vi "DCV_MultChannel.vi"(8 "Error In":errorcluster, 9 "End channel":string="116", 10 "Start channel":string="101", 11 "VISA resource name":refnum<visa-resource-name>="COM5") -> (0 "Error Out":errorcluster, 2 "testlist":dbl[](array[numeric])=[1.33831, 1.33831, 1.33831, 1.33831, 1.3383, 1.3383, 1.3383, 1.3383, 1.33829, 1.33829, 1.33829, 1.33829, 1.33828, 1.33828, 1.33828, 1.33828], 3 "VISA resource name out":refnum<visa-resource-name>="COM5")   [LabVIEW 2013]
uses:
  <vilib>/Utility/error.llb/whitespace.ctl
panel:
  out "number":dbl=1.33828
  out "read buffer":string="SCAN OK\n"
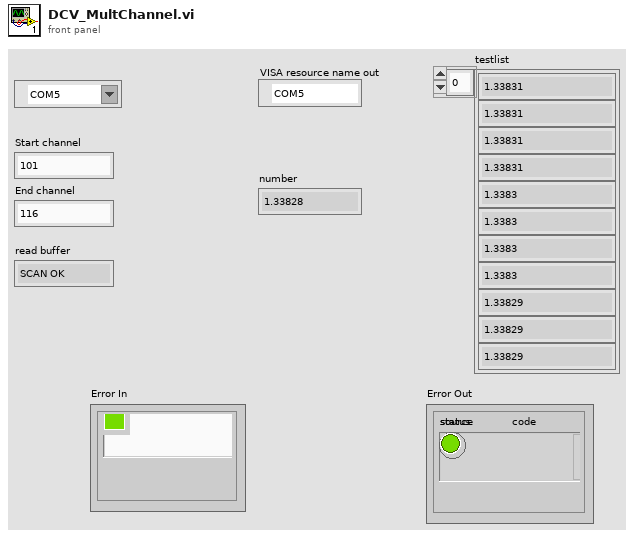
[diagram p1: front panel]
types:
  T1 = typedef "whitespace.ctl" = u16
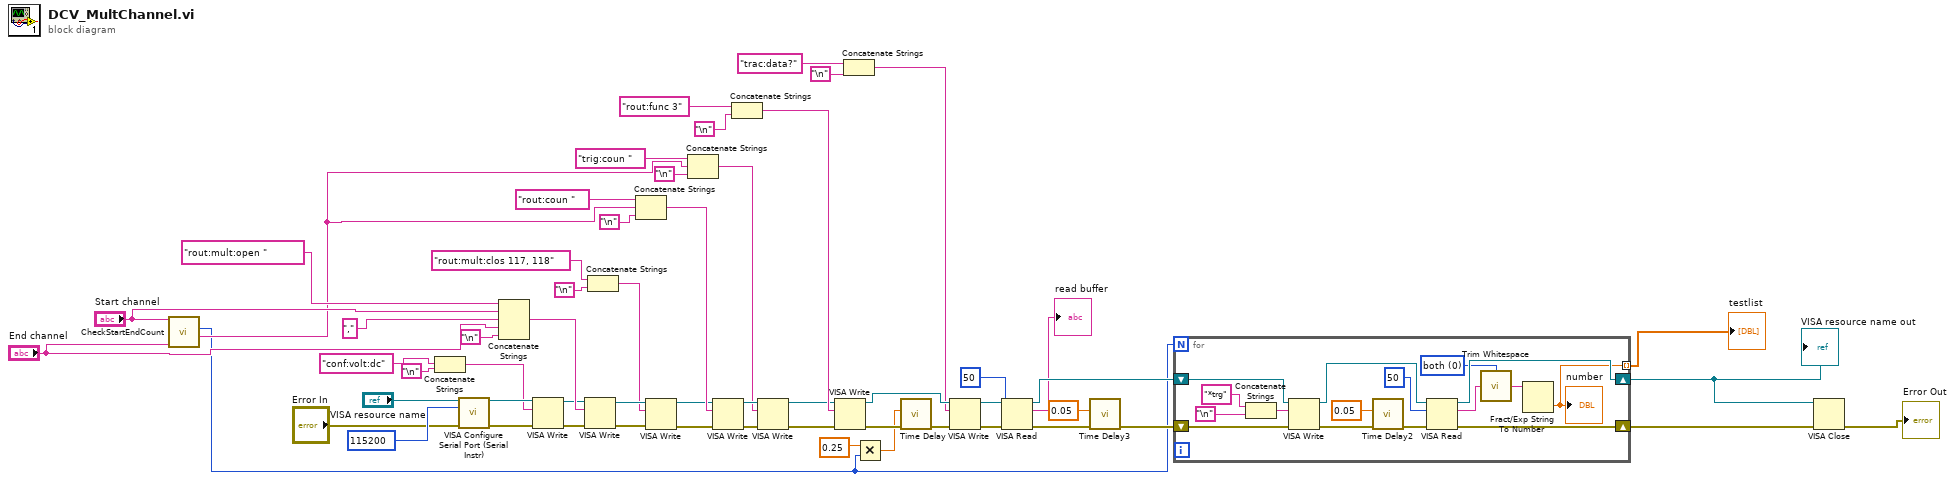
[diagram p0: block diagram]
diagram:
  n1 = call "CheckStartEndCount.vi"("End channel"="End channel", "Start channel"="Start channel") -> ("Length string"=w5:string, "Length number"=w1:i32)  [unwired: 8 in]
  n2 = Concatenate Strings("conf:volt:dc" ("write buffer"), "\n") -> (w52:string)
  n3 = call <vilib>:"VISA Configure Serial Port (Serial Instr).vi"("VISA resource name"="VISA resource name", "baud rate (9600)"=u32 115200, "error in (no error)"="Error In") -> ("VISA resource name out"=w57:refnum<visa-resource-name>, "error out"=w58:errorcluster)  [unwired: 11 in]
  n4 = Concatenate Strings("rout:mult:open ", "Start channel", ",", "End channel", "\n") -> (w48:string)
  n5 = VISA Write(VISA resource name=w57, write buffer=w52, error in (no error)=w58) -> (VISA resource name out=w47:refnum<visa-resource-name>, error out=w49:errorcluster)  [unwired: 1 out]
  n6 = VISA Write(VISA resource name=w47, write buffer=w48, error in (no error)=w49) -> (VISA resource name out=w13:refnum<visa-resource-name>, error out=w16:errorcluster)  [unwired: 1 out]
  n7 = Concatenate Strings("rout:mult:clos 117, 118" ("write buffer"), "\n") -> (w10:string)
  n8 = Concatenate Strings("rout:coun " ("write buffer"), w5, "\n") -> (w45:string)
  n9 = VISA Write(VISA resource name=w13, write buffer=w10, error in (no error)=w16) -> (VISA resource name out=w14:refnum<visa-resource-name>, error out=w15:errorcluster)  [unwired: 1 out]
  n10 = Concatenate Strings("trig:coun " ("write buffer"), w5, "\n") -> (w41:string)
  n11 = VISA Write(VISA resource name=w14, write buffer=w45, error in (no error)=w15) -> (VISA resource name out=w43:refnum<visa-resource-name>, error out=w44:errorcluster)  [unwired: 1 out]
  n12 = Concatenate Strings("rout:func 3" ("write buffer"), "\n") -> (w39:string)
  n13 = VISA Write(VISA resource name=w43, write buffer=w41, error in (no error)=w44) -> (VISA resource name out=w18:refnum<visa-resource-name>, error out=w19:errorcluster)  [unwired: 1 out]
  n14 = VISA Write(VISA resource name=w18, write buffer=w39, error in (no error)=w19) -> (VISA resource name out=w37:refnum<visa-resource-name>, error out=w38:errorcluster)  [unwired: 1 out]
  n15 = Concatenate Strings("trac:data?" ("write buffer"), "\n") -> (w27:string)
  n16 = Multiply(x=0.25, y=w1) -> (x*y=w2:dbl)
  n17 = call "Time Delay"("error in (no error)"=w38, "Delay Time (s)"=w2) -> ("error out"=w26:errorcluster)  [unwired: 9 in]
  n18 = VISA Write(VISA resource name=w37, write buffer=w27, error in (no error)=w26) -> (VISA resource name out=w24:refnum<visa-resource-name>, error out=w25:errorcluster)  [unwired: 1 out]
  n19 = VISA Read(VISA resource name=w24, byte count=u32 50, error in (no error)=w25) -> (VISA resource name out=w35:refnum<visa-resource-name>, read buffer=→"read buffer":string, error out=w21:errorcluster)  [unwired: 1 out]
  n20 = call "Time Delay3"("error in (no error)"=w21, "Delay Time (s)"=0.05) -> ("error out"=w36:errorcluster)  [unwired: 9 in]
  n21 = for {
    N: w1 -> [_]
    shift-right: [w74] -> w56
    shift-left: w36 -> [w64]
    shift-right: [w73] -> w55
    shift-left: w35 -> [w63]
    tunnel: [w59] -> w17 mode=indexing
    w61 = T1 0 items=["both", "start of string", "end of string"] ("location (both)")
    n22 = Concatenate Strings("*trg" ("write buffer"), "\n") -> (w69:string)
    n23 = VISA Write(VISA resource name=w63, write buffer=w69, error in (no error)=w64) -> (VISA resource name out=w66:refnum<visa-resource-name>, error out=w68:errorcluster)  [unwired: 1 out]
    n24 = call "Time Delay2"("error in (no error)"=w68, "Delay Time (s)"=0.05) -> ("error out"=w67:errorcluster)  [unwired: 9 in]
    n25 = VISA Read(VISA resource name=w66, byte count=u32 50, error in (no error)=w67) -> (VISA resource name out=w73:refnum<visa-resource-name>, read buffer=w62:string, error out=w74:errorcluster)  [unwired: 1 out]
    n26 = call <vilib>:"Trim Whitespace.vi"("string"=w62, "location (both)"=w61) -> ("trimmed string"=w60:string)
    n27 = Fract/Exp String To Number(string=w60) -> (number=w59:dbl)  [unwired: 3 in, 1 out]
    "number" <- w59
  }
  "VISA resource name out" <- w55
  "testlist" <- w17
  n28 = VISA Close(VISA resource name=w55, error in (no error)=w56) -> (error out=→"Error Out":errorcluster)
